vi "Build HIA command substring.vi"(2 "Axes to set":string[](array[string]), 3 "DeviceID":i32[](array[numeric]), 6 "Function":i32[](array[numeric]), 10 "DeviceAxis":string[](array[string])) -> (14 "HIA command substring":string)   [LabVIEW 2026]
doc: "This VI builds a command substring for HIA type commands. Sub-VI for HIA.vi, HIS.vi."
panel:
  # "This vi builds a command substring for HIA type commands."
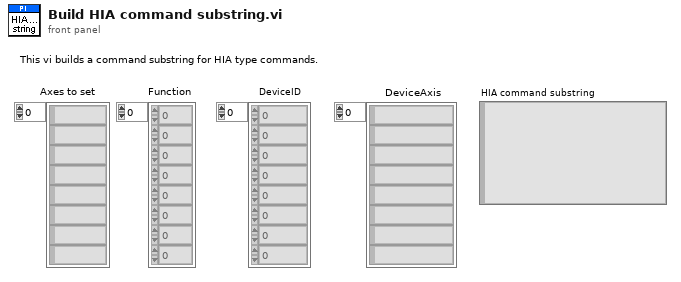
[diagram p1: front panel]
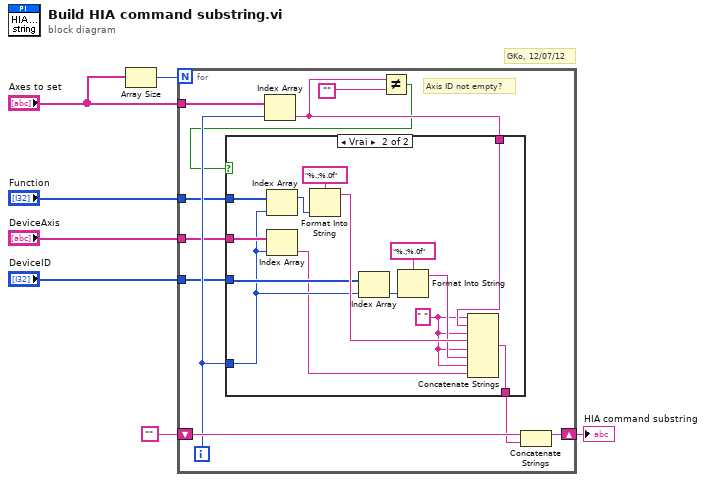
[diagram p0: block diagram]
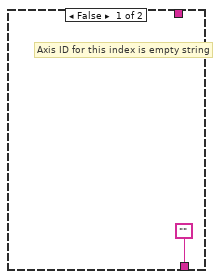
[diagram p2: hidden frame]
diagram:
  # "GKo, 12/07/12"
  n1 = Array Size(array="Axes to set") -> (size(s)=w4:i32)
  n2 = for {
    N: w4 -> [_]
    shift-right: [w17] -> w6
    shift-left: "" -> [w18]
    tunnel: "DeviceID" -> [w14]
    tunnel: "Axes to set" -> [w13]
    tunnel: "Function" -> [w9]
    tunnel: "DeviceAxis" -> [w8]
    i -> [w15]
    # "Axis ID not empty?"
    n3 = Index Array(array=w13, index=w15) -> (element=w12:string)
    n4 = Not Equal?(x=w12, y="") -> (x != y?=w10:bool)
    n5 = case shown="Vrai" w10 {
      tunnel: ["" w33] -> w16
      tunnel: w15 -> [_ w21]
      tunnel: w14 -> [_ w23]
      tunnel: w12 -> [_ w32]
      tunnel: w9 -> [_ w31]
      tunnel: w8 -> [_ w22]
      frame False {
        # "Axis ID for this index is empty string"
      }
      frame True {
        w24 = " " ("Substring")
        n6 = Index Array(array=w31, index=w21) -> (element=w29:i32)
        n7 = Index Array(array=w22, index=w21) -> (element=w20:string)
        n8 = Format Into String(format string="%.;%.0f" ("Format String"), w29) -> (resulting string=w30:string)  [unwired: 2 in, 1 out]
        n9 = Index Array(array=w23, index=w21) -> (element=w26:i32)
        n10 = Format Into String(format string="%.;%.0f" ("Format String"), w26) -> (resulting string=w25:string)  [unwired: 2 in, 1 out]
        n11 = Concatenate Strings(w24, w32, w24, w30, w24, w25, w24, w20) -> (w33:string)
      }
    }
    n12 = Concatenate Strings(w18, w16) -> (w17:string)
  }
  "HIA command substring" <- w6
